vi "Dialog_LostConnection.vi"() -> (6 "OK":bool)   [LabVIEW 2011]
panel:
  in  "stop":bool
  # "Sensor or USB cable removed\n\nCheck sensor connection \nand press OK"
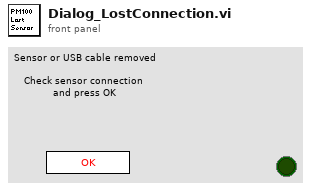
[diagram p1: front panel]
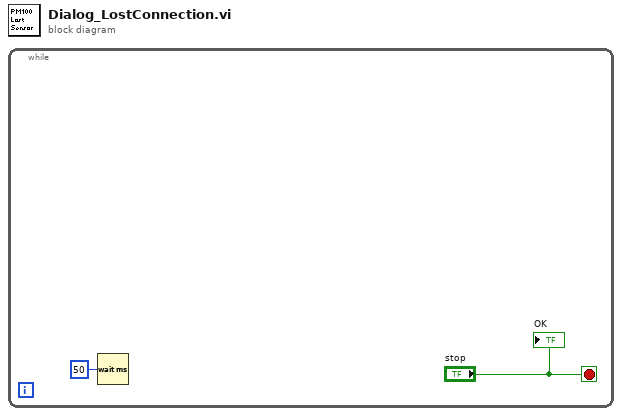
[diagram p0: block diagram]
diagram:
  n1 = while {
    stop <- "stop" stop-if-true
    n2 = Wait (ms)(milliseconds to wait=u32 50) -> ()  [unwired: 1 out]
    "OK" <- "stop"
  }
